vi "Initialize Analog IO.vi"(8 "error in":errorcluster, 11 "PLC in":refnum<class "PLC.lvclass">) -> (0 "error out":errorcluster, 3 "PLC out":refnum<class "PLC.lvclass">)   [LabVIEW 2018, in "PLC.lvlib" / "PLC.lvclass"]
uses:
  PLC.lvclass
  PLC.lvclass/PLC.ctl
  PPLs/Configuration/Configuration.lvlibp/Configuration.lvclass
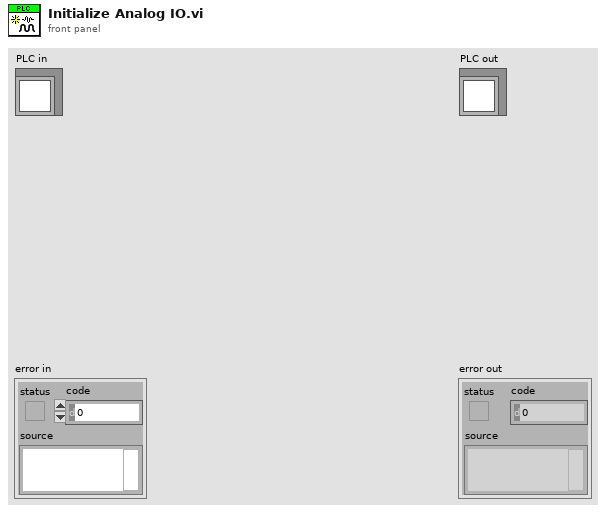
[diagram p1: front panel]
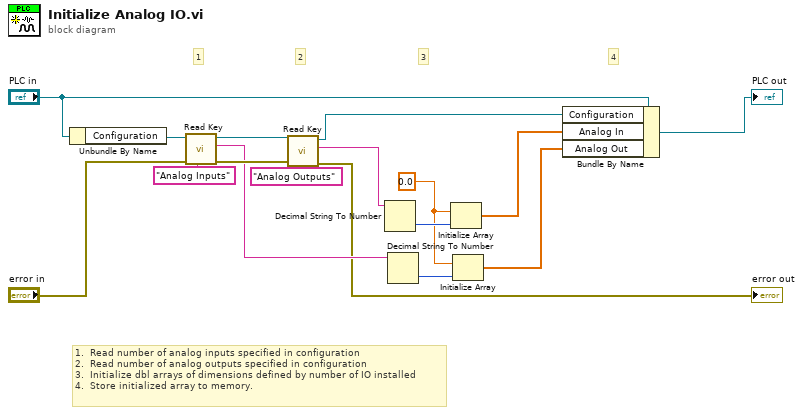
[diagram p0: block diagram]
diagram:
  w4 = 0.0
  # "4"
  # "3"
  # "2"
  # "1"
  # "1.  Read number of analog inputs specified in configuration\n2.  Read number of analog outputs specified in configuration\n3.  Initialize dbl arrays of dimensions defined by number of IO installed\n4.  Store initialized array to memory."
  n1 = Unbundle By Name("PLC in") -> ("Configuration"=w17:refnum<class "Configuration.lvclass">)
  n2 = call "Read Key.vi"("Key:"="Analog Inputs", "error in"="error in", "Configuration in"=w17) -> ("error out"=w13:errorcluster, "Value"=w7:string, "Configuration out"=w12:refnum<class "Configuration.lvclass">)  [unwired: 6 in]
  n3 = call "Read Key.vi"("Key:"="Analog Outputs", "error in"=w13, "Configuration in"=w12) -> ("error out"=→"error out":errorcluster, "Value"=w8:string, "Configuration out"=w9:refnum<class "Configuration.lvclass">)  [unwired: 6 in]
  n4 = Decimal String To Number(string=w8) -> (number=w5:i32)  [unwired: 2 in, 1 out]
  n5 = Decimal String To Number(string=w7) -> (number=w6:i32)  [unwired: 2 in, 1 out]
  n6 = Initialize Array(w4, w5) -> (w3:dbl[])
  n7 = Initialize Array(w4, w6) -> (w2:dbl[])
  n8 = Bundle By Name(cluster="PLC in", "Configuration"=w9, "Analog In"=w3, "Analog Out"=w2) -> (→"PLC out":refnum<class "PLC.lvclass">)
